vi "Comparator State.vi"(8 "error in (no error)":errorcluster, 9 "State (F: Off)":bool, 10 "Bin Count Operations (1: Off)":u32(slide)=1 max=3 step=1, 11 "VISA resource name":refnum<visa-resource-name>) -> (0 "error out":errorcluster, 3 "VISA resource name out":refnum<visa-resource-name>)   [LabVIEW 2015, in "Agilent 428X Series.lvlib"]
doc: "This function immediately sets the built_in comparator."
uses:
  Agilent 428X Series.lvlib
panel:
  # "On\nOff"
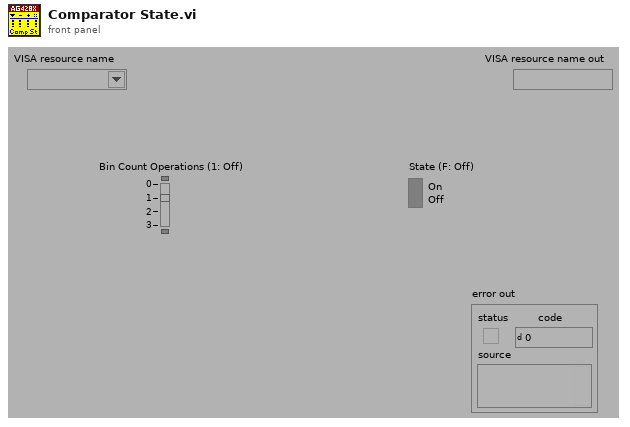
[diagram p1: front panel]
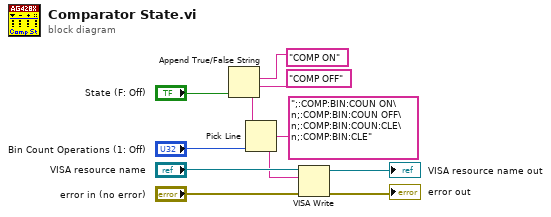
[diagram p0: block diagram]
diagram:
  n1 = Append True/False String(1:"State (F: Off)", 2:"COMP OFF", 3:"COMP ON") -> (0:w4:string)  [unwired: 1 in]
  n2 = Pick Line(string ("")=w4, multi-line string=";:COMP:BIN:COUN ON\n;:COMP:BIN:COUN OFF\n;:COMP:BIN:COUN:CLE\n;:COMP:BIN:CLE", line index="Bin Count Operations (1: Off)") -> (output string=w2:string)
  n3 = VISA Write(VISA resource name="VISA resource name", write buffer=w2, error in (no error)="error in (no error)") -> (VISA resource name out=→"VISA resource name out":refnum<visa-resource-name>, error out=→"error out":errorcluster)  [unwired: 1 out]
